vi "Check Installed.vi"(8 "error in (no error)":errorcluster, 11 "Generic Execution Adapter in":refnum<class "Generic Execution Adapter.lvclass">) -> (0 "error out":errorcluster, 1 "Message":string, 2 "Installed?":bool, 3 "Generic Execution Adapter out":refnum<class "Generic Execution Adapter.lvclass">)   [LabVIEW 2026, in "Generic Execution Adapter.lvclass"]
uses:
  Generic Execution Adapter.lvclass
  Generic Execution Adapter.lvclass/Generic Execution Adapter.ctl
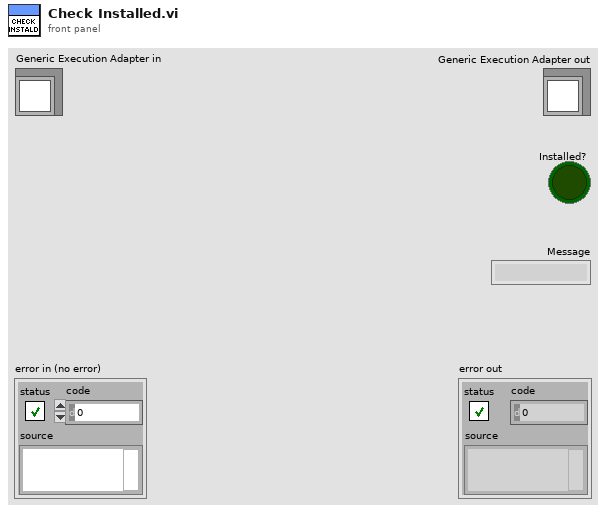
[diagram p1: front panel]
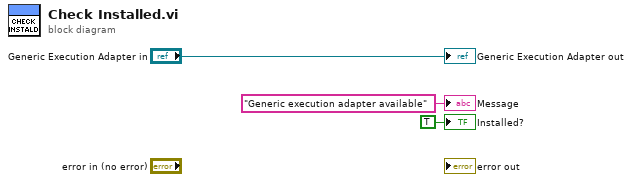
[diagram p0: block diagram]
diagram:
  "Generic Execution Adapter out" <- "Generic Execution Adapter in"
  "Message" <- "Generic execution adapter available" ("Message")
  "Installed?" <- TRUE ("Installed?")
